vi "Write DC Pins.vi"(8 "error in (no error)":errorcluster, 10 "DC Pins":string[](array[string]), 11 "Power Sweep in":refnum<class "Power Sweep.lvclass">) -> (0 "error out":errorcluster, 3 "Power Sweep out":refnum<class "Power Sweep.lvclass">)   [LabVIEW 2018, in "Power Sweep.lvlib" / "Power Sweep.lvclass"]
uses:
  Power Sweep.lvclass
  Power Sweep.lvclass/Power Sweep.ctl
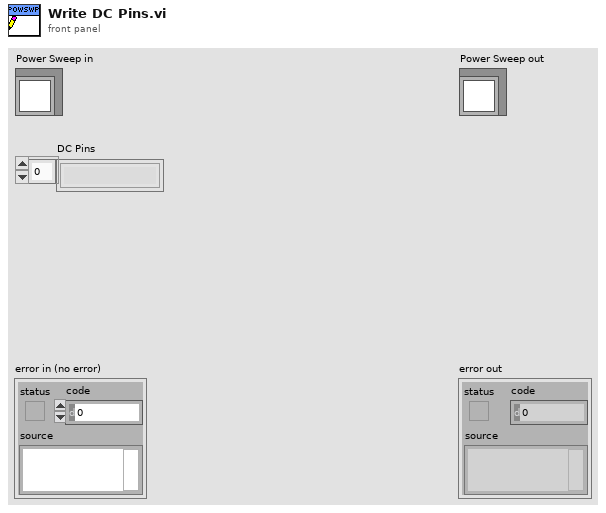
[diagram p1: front panel]
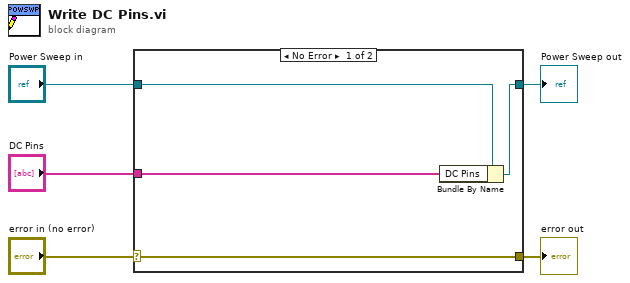
[diagram p0: block diagram]
diagram:
  n1 = case shown="No Error" "error in (no error)" {
    selector: "error in (no error)" -> [w9 w10]
    tunnel: [w9 w10] -> w4
    tunnel: [w7 w11] -> w2
    tunnel: "Power Sweep in" -> [w8 w11]
    tunnel: "DC Pins" -> [w6 _]
    frame No Error {
      n2 = Bundle By Name(cluster=w8, "DC Pins"=w6) -> (w7:refnum<class "Power Sweep.lvclass">)
    }
    frame Error {
    }
  }
  "error out" <- w4
  "Power Sweep out" <- w2
